vi "Unary ni_measurements_v1_MeasurementService_GetMetadata.vi"(8 "error in":errorcluster, 10 "Request Data":T8, 11 "gRPC ID":T9) -> (0 "error out":errorcluster, 2 "Response Data":T1, 3 "gRPC ID out":T9)   [LabVIEW 2020, in "Measurement_client.lvlib"]
uses:
  Measurement_client.lvlib
  <vilib>/gRPC/LabVIEW gRPC Library/Server API/typeDefs/grpcId.ctl
  RPC Messages/ni_measurements_v1_GetMetadataRequest.ctl
  RPC Messages/ni_measurements_v1_GetMetadataResponse.ctl
  RPC Messages/ni_measurements_v1_MeasurementDetails.ctl
  RPC Messages/ni_measurements_v1_MeasurementParameters.ctl
  RPC Messages/ni_measurements_v1_ConfigurationParameter.ctl
  RPC Messages/google_protobuf_Any.ctl
  RPC Messages/ni_measurements_v1_Output.ctl
  RPC Messages/ni_measurements_v1_UserInterfaceDetails.ctl
  3477ff3c-ac1a-41b2-98e0-1f89dff8fa77.vi
  <vilib>/gRPC/LabVIEW gRPC Library/Server API/Server/Get Server DLL Path.vi
  <vilib>/gRPC/LabVIEW gRPC Library/gprc-lvsupport-release.lvlib
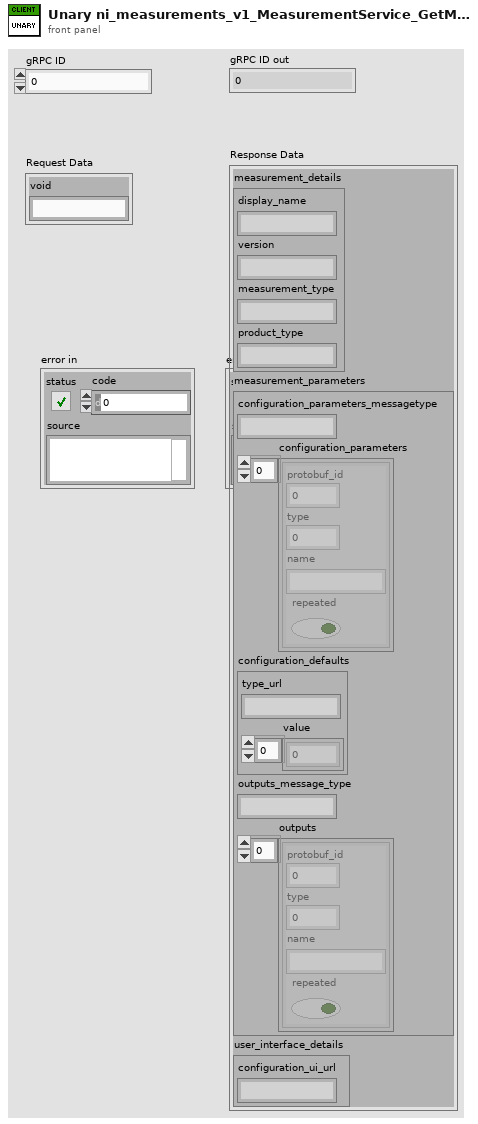
[diagram p1: front panel]
types:
  T1 = typedef "Measurement_client.lvlib/ni_measurements_v1_GetMetadataResponse.ctl" = cluster{"measurement_details":T2, "measurement_parameters":T3, "user_interface_details":T7}
  T2 = typedef "Measurement_client.lvlib/ni_measurements_v1_MeasurementDetails.ctl" = cluster{"display_name":string, "version":string, "measurement_type":string, "product_type":string}
  T3 = typedef "Measurement_client.lvlib/ni_measurements_v1_MeasurementParameters.ctl" = cluster{"configuration_parameters_messagetype":string, "configuration_parameters":T4[], "configuration_defaults":T5, "outputs_message_type":string, "outputs":T6[]}
  T4 = typedef "Measurement_client.lvlib/ni_measurements_v1_ConfigurationParameter.ctl" = cluster{"protobuf_id":u32, "type":i32, "name":string, "repeated":bool}
  T5 = typedef "Measurement_client.lvlib/google_protobuf_Any.ctl" = cluster{"type_url":string, "value":u8[]}
  T6 = typedef "Measurement_client.lvlib/ni_measurements_v1_Output.ctl" = cluster{"protobuf_id":u32, "type":i32, "name":string, "repeated":bool}
  T7 = typedef "Measurement_client.lvlib/ni_measurements_v1_UserInterfaceDetails.ctl" = cluster{"configuration_ui_url":string}
  T8 = typedef "Measurement_client.lvlib/ni_measurements_v1_GetMetadataRequest.ctl" = cluster{"void":string}
  T9 = typedef "gprc-lvsupport-release.lvlib/grpcId.ctl" = u64
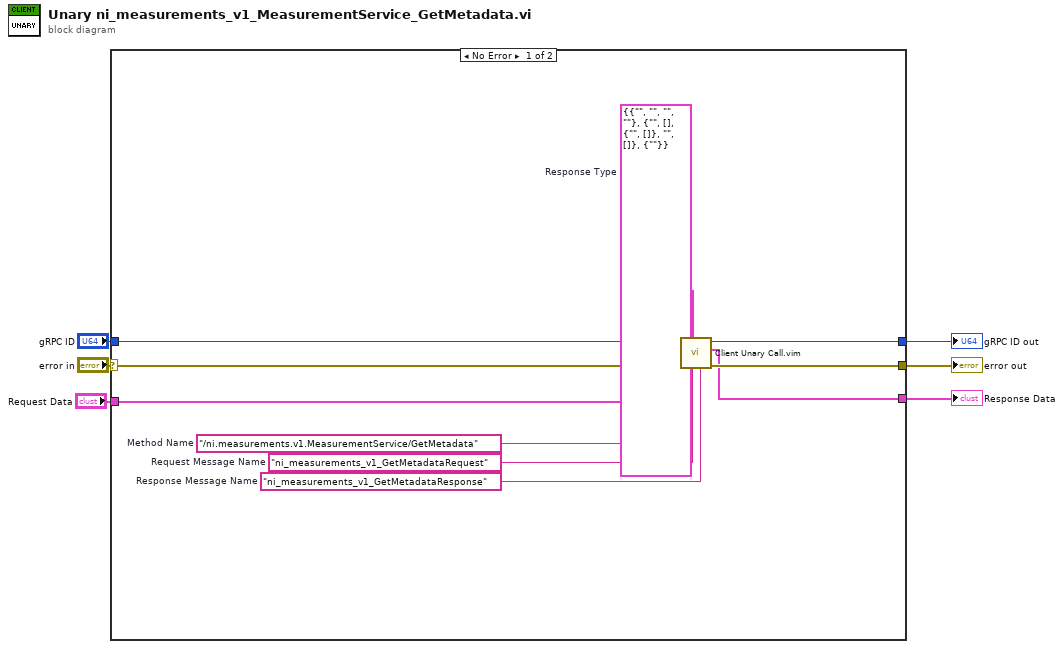
[diagram p0: block diagram]
diagram:
  n1 = case shown="No Error" "error in" {
    selector: "error in" -> [w12 w17]
    tunnel: [w11 w17] -> w5
    tunnel: "gRPC ID" -> [w10 w18]
    tunnel: [w9 w18] -> w3
    tunnel: "Request Data" -> [w8 _]
    tunnel: [w7 _] -> w1
    frame No Error {
      w13 = "ni_measurements_v1_GetMetadataResponse"  # Response Message Name
      w14 = "ni_measurements_v1_GetMetadataRequest"  # Request Message Name
      w15 = T1 {"measurement_details"={"display_name"="", "version"="", "measurement_type"="", "product_type"=""}, "measurement_parameters"={"configuration_parameters_messagetype"="", "configuration_parameters"=[], "configuration_defaults"={"type_url"="", "value"=[]}, "outputs_message_type"="", "outputs"=[]}, "user_interface_details"={"configuration_ui_url"=""}}  # Response Type
      w16 = "/ni.measurements.v1.MeasurementService/GetMetadata"  # Method Name
      n2 = call "Client Unary Call.vim"("Response Message Name"=w13, "Request Message Name"=w14, "Response Type"=w15, "error in (no error)"=w12, "Request Data"=w8, "Method Name"=w16, "Client Ref"=w10) -> ("error out"=w11:errorcluster, "Response Data"=w7:T1, "Client Ref Out"=w9:u64)  [unwired: 2 in]
    }
    frame Error {
    }
  }
  "error out" <- w5
  "gRPC ID out" <- w3
  "Response Data" <- w1
